vi "ICM Write General Parameters.vi"(8 "error out 2":errorcluster, 9 "Re-Init?":bool, 10 "ICM File In":path, 11 "ICM General Parameters":T1 {"Time" format="%<%H:%M:%S>t"; "Date" format="%<%Y/%m/%d>T"; "Version" format="%.1g"}) -> (0 "error out":errorcluster)   [LabVIEW 2018]
doc: "ICM Write General Parameters.vi\n\nThis VI is used to write the General Parameters to the ICM Configuration file.\n\nInstrument Communication Module Version 1.0\nAugust, 2017 Original Code Consulting David Thomson\n www.originalcode.com"
uses:
  ICM General Parameters.ctl
panel:
  # "The values for these\nparameters are generally\nset by the ICM system and\nneed not be edited directly."
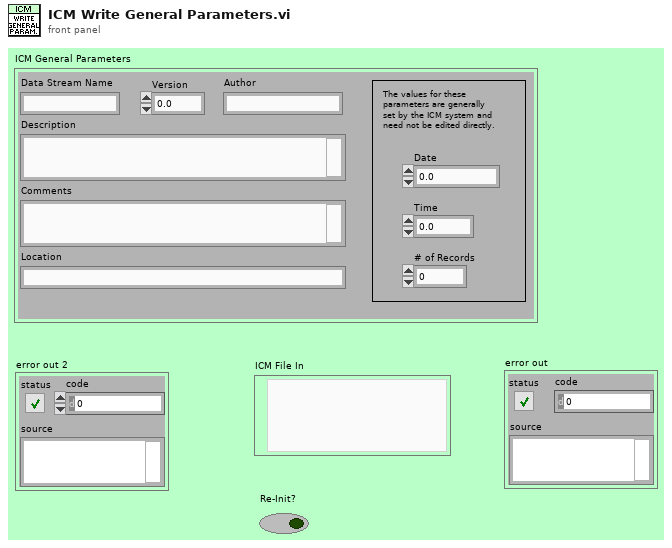
[diagram p1: front panel]
types:
  T1 = typedef "ICM General Parameters.ctl" = cluster{"Data Stream Name":string, "Version":sgl, "Author":string, "Description":string, "Comments":string, "Date":dbl, "Time":dbl, "Location":string, "# of Records":i32}
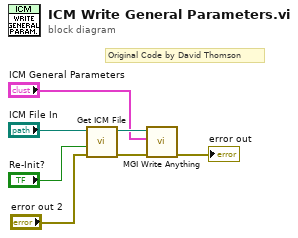
[diagram p0: block diagram]
diagram:
  # "Original Code by David Thomson"
  n1 = call "Get ICM File.vi"("error in (no error)"="error out 2", "Re-Init?"="Re-Init?", "ICM File In"="ICM File In") -> ("error out"=w7:errorcluster, "ICM File"=w6:path)  [unwired: 7 in]
  n2 = call "MGI Write Anything.vi"("Error In"=w7, "Anything"="ICM General Parameters", "Path (dialog)"=w6) -> ("Error Out"=→"error out":errorcluster)  [unwired: 6 in, 2 out]
